vi "Deadband.vi"(8 "Value to Deadband (default of 0.1)":dbl, 11 "Value":dbl) -> (3 "Deadbanded Value":dbl)   [LabVIEW 2012]
panel:
  # "Used more than once at a time,\ntherefore VI Properties > Execution\nshould be Preallocated clone reentrant"
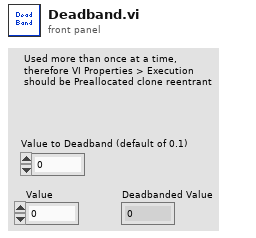
[diagram p1: front panel]
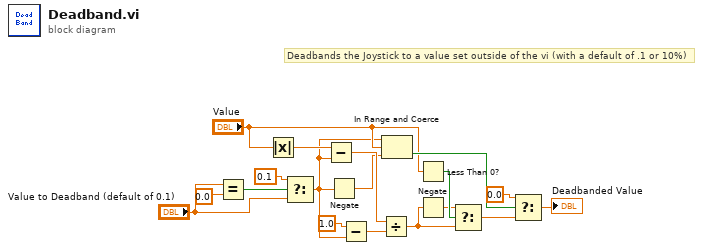
[diagram p0: block diagram]
diagram:
  # "Deadbands the Joystick to a value set outside of the vi (with a default of .1 or 10%)"
  n1 = Equal?(x="Value to Deadband (default of 0.1)", y=0.0) -> (x = y?=w4:bool)
  n2 = Absolute Value(x="Value") -> (abs(x)=w16:dbl)
  n3 = Select(t=0.1, s=w4, f="Value to Deadband (default of 0.1)") -> (s? t:f=w5:dbl)
  n4 = Subtract(x=w16, y=w5) -> (x-y=w15:dbl)
  n5 = Negate(x=w5) -> (-x=w8:dbl)
  n6 = Subtract(x=1.0, y=w5) -> (x-y=w6:dbl)
  n7 = Divide(x=w15, y=w6) -> (x/y=w12:dbl)
  n8 = In Range and Coerce(upper limit=w5, x="Value", lower limit=w8) -> (In Range?=w18:bool)  [unwired: 1 out]
  n9 = Less Than 0?(x="Value") -> (x < 0?=w14:bool)
  n10 = Negate(x=w12) -> (-x=w13:dbl)
  n11 = Select(t=w13, s=w14, f=w12) -> (s? t:f=w10:dbl)
  n12 = Select(t=0.0, s=w18, f=w10) -> (s? t:f=→"Deadbanded Value":dbl)
